vi "read.vi"() -> ()   [LabVIEW 2025]
uses:
  <vilib>/sound2/lvsound2.llb/Sound Data Format.ctl
  <vilib>/sound2/lvsound2.llb/Sound File Info (path).vi
panel:
  out "sound format":T1={"sample rate (S/s)"=22050.0, "number of channels"=2, "bits per sample"=16}
  out "1/x":dbl
  out "dt":dbl
  out "Salida de Audio":waveform(dbl)(graph)
  out "Entrada de Audio":waveform(dbl)(graph)
  in  "Output":path
  in  "Input":path
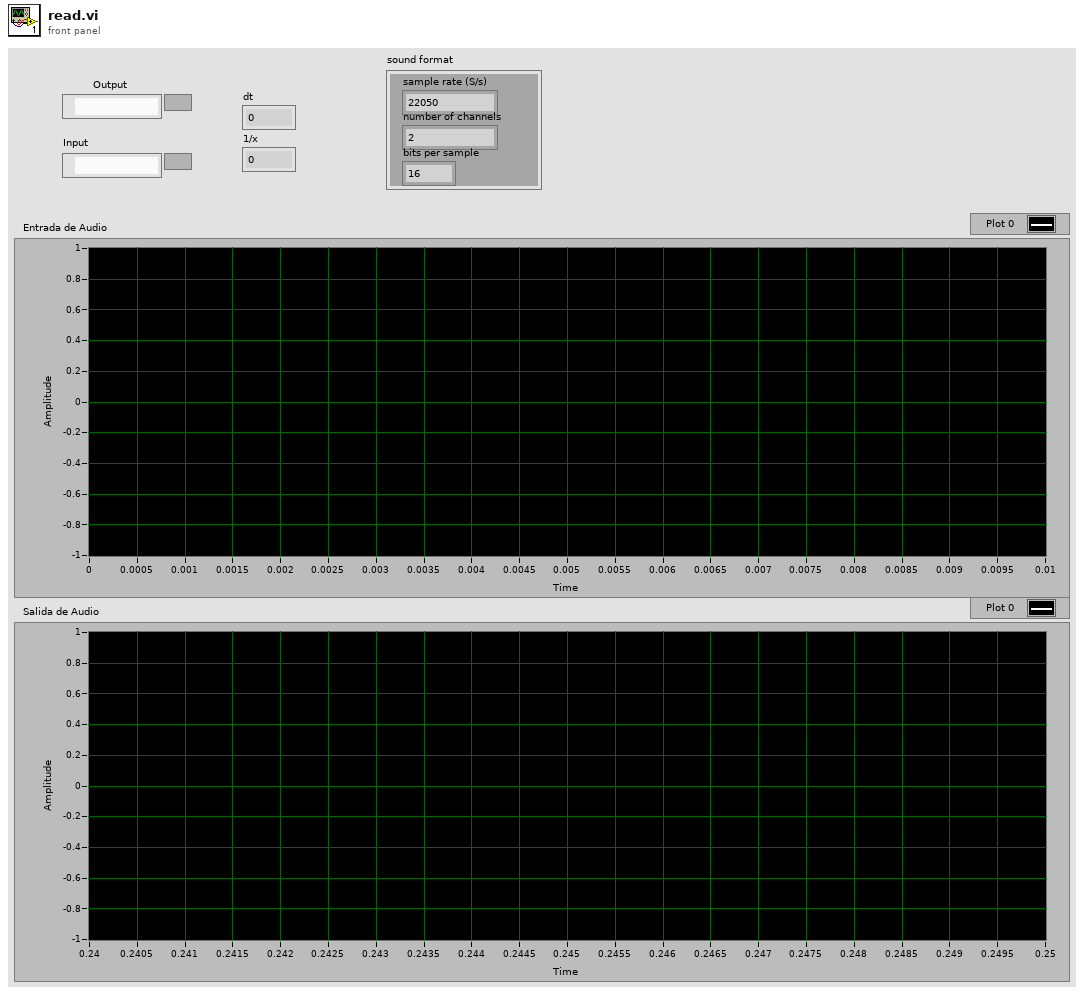
[diagram p1: front panel]
types:
  T1 = typedef "Sound Data Format.ctl" = cluster{"sample rate (S/s)":dbl, "number of channels":i32, "bits per sample":i32}
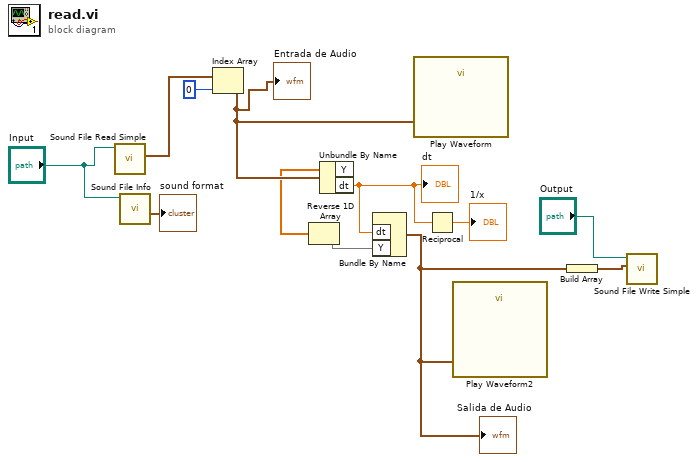
[diagram p0: block diagram]
diagram:
  n1 = call <vilib>:"Sound File Read Simple.vi"("path"="Input") -> ("data"=w12:waveform(dbl)[])  [unwired: 7 in, 3 out]
  n2 = call-poly <vilib>:"Sound File Info.vi"("path"="Input") -> ("sound format"=→"sound format":T1)  [unwired: 7 in, 3 out]
  n3 = Index Array(array=w12, index=0) -> (element=w10:waveform(dbl))
  "Entrada de Audio" <- w10
  n4 = Unbundle By Name(w10) -> ("Y"=w4:dbl[], "dt"=w6:dbl)
  "dt" <- w6
  n5 = Reverse 1D Array(array=w4) -> (reversed array=w5:dbl[])
  n6 = Bundle By Name("dt"=w6, "Y"=w5) -> (w2:waveform(dbl))  [unwired: 1 in]
  "Salida de Audio" <- w2
  n7 = call "Play Waveform"("Data"=w10) -> ()  [unwired: 18 in, 1 out]
  n8 = Reciprocal(x=w6) -> (1/x=→"1/x":dbl)
  n9 = call "Play Waveform2"("Data"=w2) -> ()  [unwired: 18 in, 1 out]
  n10 = Build Array(w2) -> (w3:waveform(dbl)[])
  n11 = call <vilib>:"Sound File Write Simple.vi"("data"=w3, "path"="Output") -> ()  [unwired: 8 in, 2 out]
